vi "Prompt Reset.vi"(8 "error in (no error)":errorcluster, 11 "RP2040Target in":refnum<class "RP2040Target.lvclass">) -> (0 "error out":errorcluster, 3 "RP2040Target out":refnum<class "RP2040Target.lvclass">)   [LabVIEW 2020, in "RP2040.lvlib" / "RP2040Target.lvclass"]
uses:
  RP2040Target.lvclass
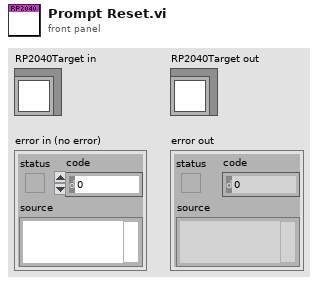
[diagram p1: front panel]
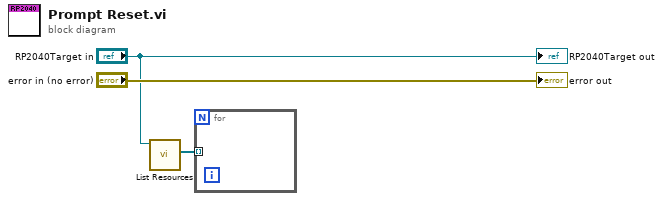
[diagram p0: block diagram]
diagram:
  n1 = call-dynamic "List Resources.vi"("RP2040Target in"="RP2040Target in") -> ("Resources"=w2:refnum<class "DeployResource.lvclass">[])  [unwired: 8 in, 2 out]
  n2 = for {
    tunnel: w2 -> [_] mode=indexing
  }
  "error out" <- "error in (no error)"
  "RP2040Target out" <- "RP2040Target in"
